vi "Simple Clock Gen And Bus Monitor.vi"() -> ()   [LabVIEW 2021, in "IO.lvclass"]
uses:
  IO.lvclass
  <vilib>/DAQmx/write.llb/DAQmx Write (Digital Bool 1Line 1Point).vi
  <vilib>/DAQmx/read.llb/DAQmx Read (Digital Bool 1Line 1Point).vi
  <vilib>/DAQmx/read.llb/DAQmx Read (Digital 1D Bool NChan 1Samp 1Line).vi
  <vilib>/DAQmx/miscellaneous.llb/DAQmx Fill In Error Info.vi
  <resource>/objmgr/daqmx.rc
panel:
  out "R/W":bool
  out "Data":u8 format="%04x"
  out "Data":bool[](array[boolean])
  in  "CLK":bool
  out "Address":u16 format="%04x"
  out "Address":bool[](array[boolean])
  # "Clock rising edge: setup data\n\nClock falling edge: sample data"
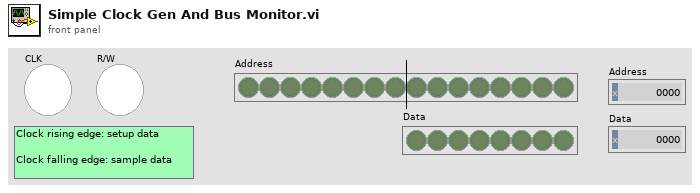
[diagram p1: front panel]
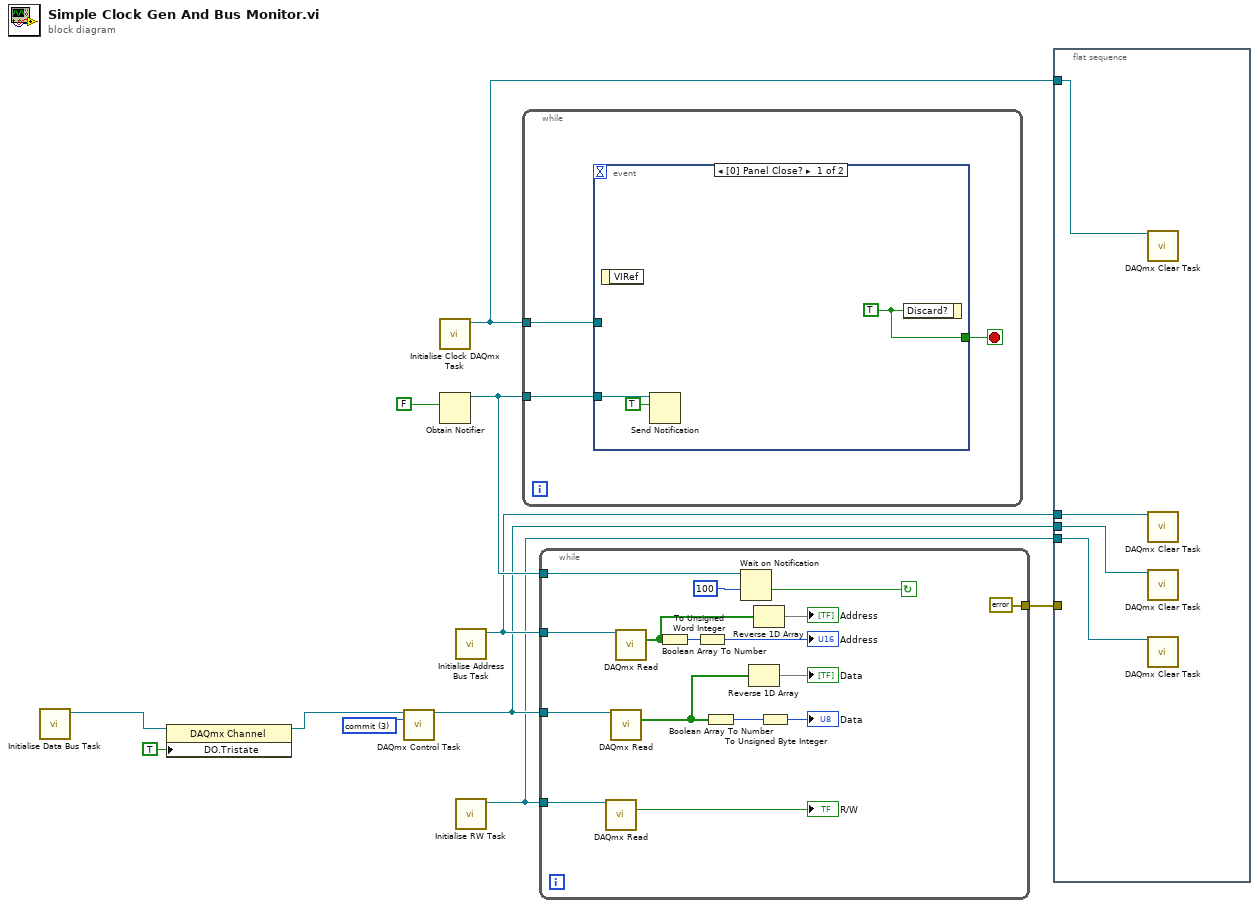
[diagram p0: block diagram]
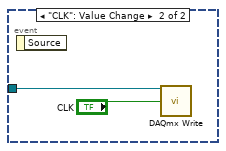
[diagram p2: hidden frame]
diagram:
  w11 = 3 items=["verify"=2, "reserve"=4, "commit"=3, "unreserve"=5, "abort"=6] ("action")
  n1 = call "Initialise Data Bus Task.vi"() -> ("Data Bus"=w8:refnum<k21>)  [unwired: 10 in, 1 out]
  n2 = property class="DAQmx Channel"(reference=w8, "DO.Tristate"=TRUE) -> (reference out=w10:refnum<k21>)  [unwired: 1 in, 1 out]
  n3 = call <vilib>:"DAQmx Control Task.vi"("task/channels in"=w10, "action"=w11) -> ("task out"=w2:refnum<k21>)  [unwired: 12 in, 1 out]
  n4 = call "Initialise Clock DAQmx Task.vi"() -> ("task out"=w4:refnum<k21>)  [unwired: 10 in, 1 out]
  n5 = Obtain Notifier(notification data type=FALSE) -> (notifier out=w6:refnum<notifier>)  [unwired: 3 in, 2 out]
  n6 = call "Initialise Address Bus Task.vi"() -> ("Address Bus"=w3:refnum<k21>)  [unwired: 10 in, 1 out]
  n7 = call "Initialise RW Task.vi"() -> ("R/W"=w1:refnum<k21>)  [unwired: 10 in, 1 out]
  n8 = while {
    tunnel: w4 -> [w13]
    tunnel: w6 -> [w12]
    stop <- w14 stop-if-true
    n9 = event shown="[0] Panel Close?" {
      selector: _ -> [_ _]
      dyn-events: _ -> [_ _]
      timeout: _ -> [_ _]
      tunnel: [w18 _] -> w14
      tunnel: w13 -> [w17 w19]
      tunnel: [w17 _] -> _
      tunnel: w12 -> [w16 _]
      event Panel Close? {
        w18 = TRUE ("Discard?")
        n10 = event-data() -> ()  [unwired: 1 in, 1 out]
        n11 = Send Notification(notification=TRUE, notifier=w16) -> ()  [unwired: 1 in, 2 out]
        n12 = event-data("Discard?"=w18) -> ()  [unwired: 1 in, 1 out]
      }
      event "CLK": Value Change {
        n13 = event-data() -> ()  [unwired: 1 in, 1 out]
        n14 = call-poly <vilib>:"DAQmx Write.vi"("task/channels in"=w19, "data"="CLK") -> ()  [unwired: 11 in, 3 out]
      }
    }
  }
  n15 = while {
    tunnel: w3 -> [w35]
    tunnel: w2 -> [w32]
    tunnel: w1 -> [w30]
    tunnel: w6 -> [w28]
    tunnel: [errorcluster {"status"=FALSE, "code"=0, "source"=""} ("error constant")] -> w5
    stop <- w26 continue-if-true
    n16 = call-poly <vilib>:"DAQmx Read.vi"("task/channels in"=w30) -> ("data"=→"R/W":bool)  [unwired: 12 in, 2 out]
    n17 = call-poly <vilib>:"DAQmx Read.vi"("task/channels in"=w32) -> ("data"=w22:bool[])  [unwired: 12 in, 2 out]
    n18 = call-poly <vilib>:"DAQmx Read.vi"("task/channels in"=w35) -> ("data"=w24:bool[])  [unwired: 12 in, 2 out]
    n19 = Boolean Array To Number(Boolean array=w24) -> (number=w36:u32)
    n20 = To Unsigned Word Integer(number=w36) -> (unsigned 16bit integer=→"Address":u16)
    n21 = Boolean Array To Number(Boolean array=w22) -> (number=w33:u32)
    n22 = Wait on Notification(notifier=w28, timeout in ms (-1)=u32 100 ("milliseconds to wait")) -> (timed out?=w26:bool)  [unwired: 2 in, 3 out]
    n23 = Reverse 1D Array(array=w22) -> (reversed array=→"Data":bool[])
    n24 = Reverse 1D Array(array=w24) -> (reversed array=→"Address":bool[])
    n25 = To Unsigned Byte Integer(number=w33) -> (unsigned 8bit integer=→"Data":u8)
  }
  n26 = flat-sequence {
    tunnel: w5 -> [_]
    tunnel: w4 -> [w40]
    tunnel: w3 -> [w39]
    tunnel: w2 -> [w38]
    tunnel: w1 -> [w37]
    frame #0 {
      n27 = call <vilib>:"DAQmx Clear Task.vi"("task in"=w40) -> ()  [unwired: 14 in, 1 out]
      n28 = call <vilib>:"DAQmx Clear Task.vi"("task in"=w39) -> ()  [unwired: 14 in, 1 out]
      n29 = call <vilib>:"DAQmx Clear Task.vi"("task in"=w38) -> ()  [unwired: 14 in, 1 out]
      n30 = call <vilib>:"DAQmx Clear Task.vi"("task in"=w37) -> ()  [unwired: 14 in, 1 out]
    }
  }
